vi "GoogleMapsAPI_V2009.vi"() -> ()   [LabVIEW 2015]
panel:
  in  "Color":string(combo)
  in  "Home Char":string
  in  "stop":bool
  in  "Show Path?":bool=TRUE
  in  "Weight":i32=5
  in  "Path Collor":u32(colorbox)=16715776
  in  "character":string="a"
  in  "color":string(combo)="purple"
  in  "Longitude":dbl=-1.307 format="%#.6g"
  in  "Latitude":dbl=51.4062 format="%#.6g"
  in  "Map Format":string(combo)="hybrid"
  in  "X":dbl=350.0
  in  "Y":dbl=570.0
  in  "Zoom":sgl=18.0 format="%#.1g"
  in  "Lontitude_Home":dbl=-1.3070000000000026 format="%#.6g"
  in  "Latitude_Home":dbl=51.4062 format="%#.6g"
  out "URL":string="http://maps.google.com/staticmap?center=51.406200,-1.307000&zoom=18&size=570x350&maptype=hybrid&markers=51.406200,-1.307000,midpurplea&key=&path=rgb:0xFF1000,weight:5|51.406200,-1.307000|51.406200,-1.307000"
  in  "?":refnum<k7>(container)
  # "Home Position"
  # "QuadRotor Position"
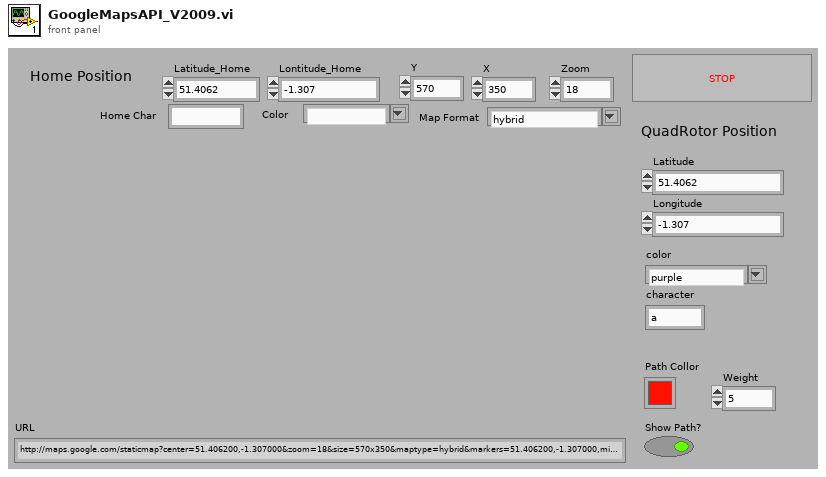
[diagram p1: front panel]
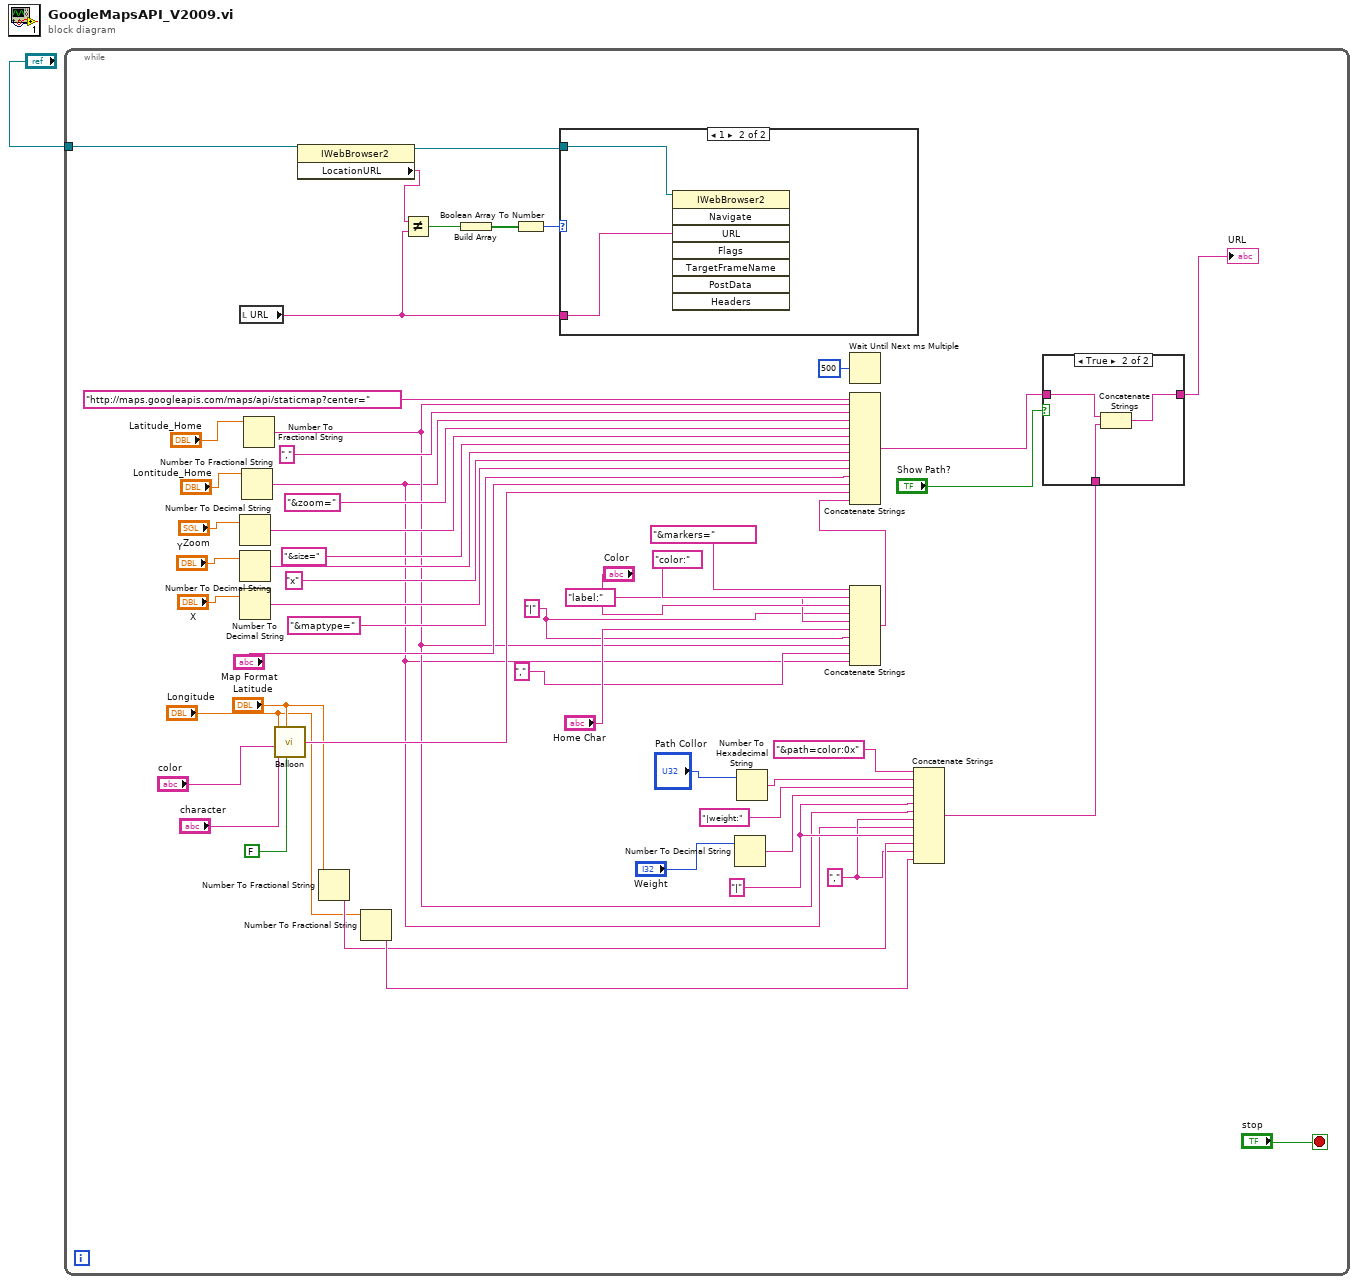
[diagram p0: block diagram]
diagram:
  n1 = while {
    tunnel: "?" -> [w54]
    stop <- "stop" stop-if-true
    w7 = "|"
    w16 = "," ("string")
    w17 = "|"
    n2 = local read "URL"() -> (w48:string)
    n3 = Number To Decimal String(number="Zoom") -> (decimal integer string=w41:string)  [unwired: 1 in]
    n4 = Number To Decimal String(number="Y") -> (decimal integer string=w37:string)  [unwired: 1 in]
    n5 = Number To Decimal String(number="X") -> (decimal integer string=w35:string)  [unwired: 1 in]
    n6 = Number To Fractional String(number="Lontitude_Home") -> (F-format string=w4:string)  [unwired: 3 in]
    n7 = Number To Fractional String(number="Latitude_Home") -> (F-format string=w5:string)  [unwired: 3 in]
    n8 = call "Balloon.vi"("One more?"=FALSE, "Latitude"="Latitude", "character"="character", "color"="color", "Longitude"="Longitude") -> ("Balloon"=w32:string)  [unwired: 1 in]
    n9 = property class="IWebBrowser2"(reference=w54) -> (reference out=w53:refnum<k7>, "LocationURL"=w51:string)  [unwired: 1 in, 1 out]
    n10 = Number To Fractional String(number="Latitude") -> (F-format string=w18:string)  [unwired: 3 in]
    n11 = Number To Fractional String(number="Longitude") -> (F-format string=w19:string)  [unwired: 3 in]
    n12 = Not Equal?(x=w51, y=w48) -> (x != y?=w52:bool)
    n13 = Build Array(w52) -> (w50:bool[])
    n14 = Boolean Array To Number(Boolean array=w50) -> (number=w49:u32)
    n15 = case shown="1" w49 {
      tunnel: w48 -> [_ w61]
      tunnel: w53 -> [_ w60]
      frame 0, Default {
      }
      frame 1 {
        n16 = invoke class="IWebBrowser2" method="Navigate"(reference=w60, "URL"=w61) -> ()  [unwired: 6 in, 8 out]
      }
    }
    n17 = Number To Decimal String(number="Weight") -> (decimal integer string=w23:string)  [unwired: 1 in]
    n18 = Number To Hexadecimal String(2:"Path Collor") -> (0:w26:string)  [unwired: 1 in]
    n19 = Wait Until Next ms Multiple(millisecond multiple=u32 500) -> ()  [unwired: 1 out]
    n20 = Concatenate Strings("&markers=", "color:", "Color", w7, "label:", "Home Char", w7, w5, ",", w4) -> (w3:string)
    n21 = Concatenate Strings("http://maps.googleapis.com/maps/api/staticmap?center=" ("URL"), w5, "," ("string"), w4, "&zoom=", w41, "&size=", w37, "x", w35, "&maptype=", "Map Format", w32, w3) -> (w20:string)
    n22 = Concatenate Strings("&path=color:0x" ("string"), w26, "|weight:", w23, w17, w5, w16, w4, w17, w18, w16, w19) -> (w2:string)
    n23 = case shown="True" "Show Path?" {
      tunnel: w2 -> [_ w59]
      tunnel: [w56 w58] -> w21
      tunnel: w20 -> [w56 w57]
      frame False {
      }
      frame True {
        n24 = Concatenate Strings(w57, w59) -> (w58:string)
      }
    }
    "URL" <- w21
  }
